vi "Decode Topic Subscriptions.vi"(10 "Payload":u8[](array[numeric]) format="%08b") -> (0 "invalid UTF8":bool, 1 "Valid?":bool, 2 "Topic Subscriptions":T1[](array[typedef]))   [LabVIEW 2013, in "SUBSCRIBE.lvclass"]
uses:
  SUBSCRIBE.lvclass
  Topic Subscription -- cluster.ctl
  ControlPacket/QualityOfService -- enum.ctl
  ControlPacket/ControlPacket.lvclass
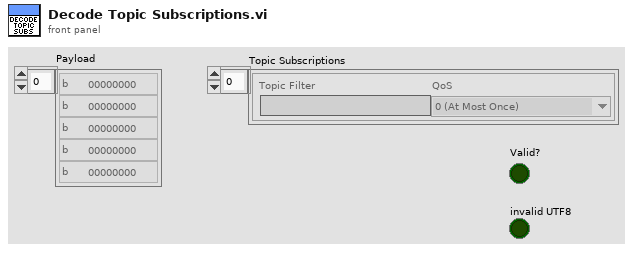
[diagram p1: front panel]
types:
  T1 = typedef "SUBSCRIBE.lvclass/Topic Subscription -- cluster.ctl" = cluster{"Topic Filter":string, "QoS":T2}
  T2 = typedef "ControlPacket.lvclass/QualityOfService -- enum.ctl" = enum16{"0 (At Most Once)", "1 (At Least Once)", "2 (Exactly Once)"}
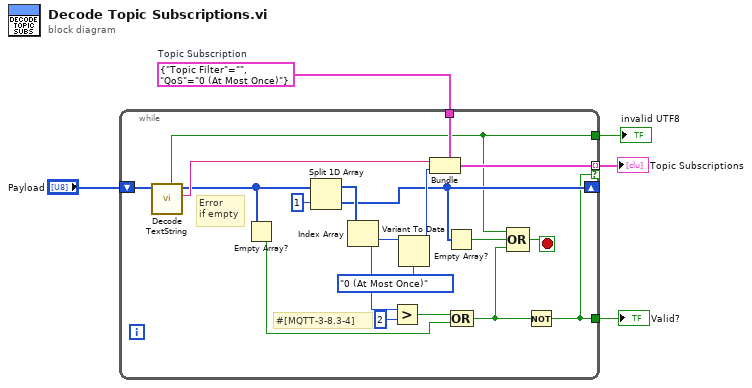
[diagram p0: block diagram]
diagram:
  w4 = T1 {"Topic Filter"="", "QoS"=enum."0 (At Most Once)"}  # Topic Subscription
  n1 = while {
    shift-right: [w16] -> _
    shift-left: "Payload" -> [w24]
    tunnel: w4 -> [w18]
    tunnel: [w17] -> w3 mode=indexing if=w7
    tunnel: [w7] -> w2
    tunnel: [w6] -> w1
    stop <- w8 stop-if-true
    # "#[MQTT-3-8.3-4]"
    # "Error\nif empty"
    n2 = call "Decode TextString.vi"("Length-Prefixed Field"=w24) -> ("Text String"=w19:string, "Remaining Packets"=w15:u8[], "restricted code"=w6:bool)  [unwired: 8 in]
    n3 = Empty Array?(array=w15) -> (empty?=w11:bool)
    n4 = Split 1D Array(array=w15, index=1) -> (first subarray=w22:u8[], second subarray=w16:u8[])
    n5 = Index Array(array=w22) -> (element=w14:u8)  [unwired: 1 in]
    n6 = Greater?(x=w14, y=u8 2) -> (0:w12:bool)
    n7 = Variant To Data(type=QualityOfService_--_enum."0 (At Most Once)" ("QoS"), Variant=w14) -> (data=w20:T2)  [unwired: 1 in, 1 out]
    n8 = Bundle(cluster=w18, "Topic Filter"=w19, "QoS"=w20) -> (w17:T1)
    n9 = Empty Array?(array=w16) -> (empty?=w9:bool)
    n10 = Compound Arithmetic op=OR(w12, w11) -> (w10:bool)
    n11 = Compound Arithmetic op=OR(w6, w9, w10) -> (w8:bool)
    n12 = Not(x=w10) -> (.not. x?=w7:bool)
  }
  "Topic Subscriptions" <- w3
  "Valid?" <- w2
  "invalid UTF8" <- w1
